vi "arduinoTest.vi"() -> ()   [LabVIEW 2019]
panel:
  out "Timed Out":bool[](array[boolean])
  in  "Commands to Send":T1(array[cluster])=[{"Command"="ST", "Wait For Completion"=TRUE, "Description"="Get status", "Timeout (ms)"=3000.0}, {"Command"="HE", "Wait For Completion"=TRUE, "Description"="Get help", "Timeout (ms)"=3000.0}, {"Command"="CW", "Wait For Completion"=TRUE, "Description"="Get current well", "Timeout (ms)"=3000.0}, {"Command"="FK", "Wait For Completion"=TRUE, "Description"="Bad command to test timeout", "Timeout (ms)"=3000.0}, {"Command"="PSx", "Wait For Completion"=TRUE, "Description"="Get x-axis position", "Timeout (ms)"=3000.0}, {"Command"="PSy", "Wait For Completion"=TRUE, "Description"="get y-axis position", "Timeout (ms)"=3000.0}, {"Command"="TM", "Wait For Completion"=TRUE, "Description"="Test Motor", "Timeout (ms)"=30000.0}, {"Command"="ST", "Wait For Completion"=TRUE, "Description"="Check status", "Timeout (ms)"=3000.0}, {"Command"="FW", "Wait For Completion"=TRUE, "Description"="Gi to first well", "Timeout (ms)"=3000.0}, {"Command"="MO", "Wait For Completion"=TRUE, "Description"="Move to next well", "Timeout (ms)"=3000.0}, {"Command"="ABX1000", "Wait For Completion"=TRUE, "Description"="Absolute move", "Timeout (ms)"=3000.0}, {"Command"="ABY1000", "Wait For Completion"=TRUE, "Description"="Test Motor", "Timeout (ms)"=3000.0}, {"Command"="ABZ1000", "Wait For Completion"=TRUE, "Description"="Test Motor", "Timeout (ms)"=3000.0}, {"Command"="REX1000", "Wait For Completion"=TRUE, "Description"="Test Motor", "Timeout (ms)"=3000.0}, {"Command"="REY1000", "Wait For Completion"=TRUE, "Description"="Test Motor", "Timeout (ms)"=3000.0}, {"Command"="REZ2000", "Wait For Completion"=TRUE, "Description"="Test Motor", "Timeout (ms)"=3000.0}]
  out "Commands Accepted":bool[](array[boolean])
  in  "Wait For Startup (ms)":u32=10000
  out "Recieve Log":string
  out "error out":errorcluster
  in  "Baud Rate":u32=9600
  in  "COM Port":refnum<visa-resource-name>="COM4"
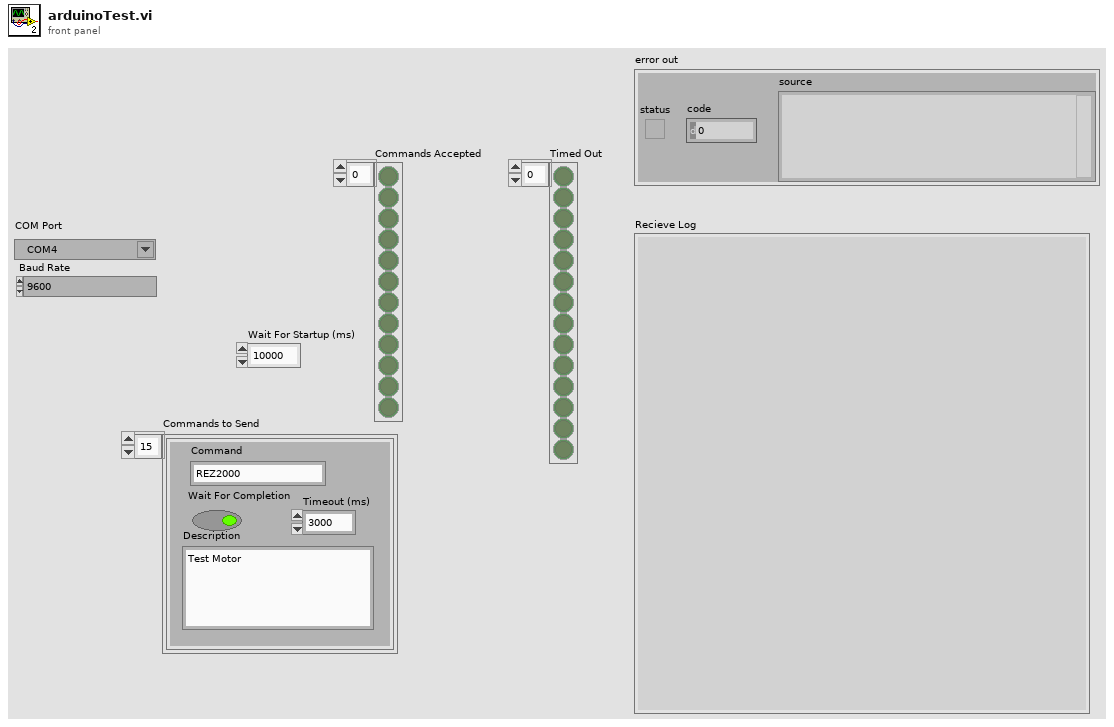
[diagram p1: front panel]
types:
  T1 = cluster{"Command":string, "Wait For Completion":bool, "Description":string, "Timeout (ms)":dbl}[]
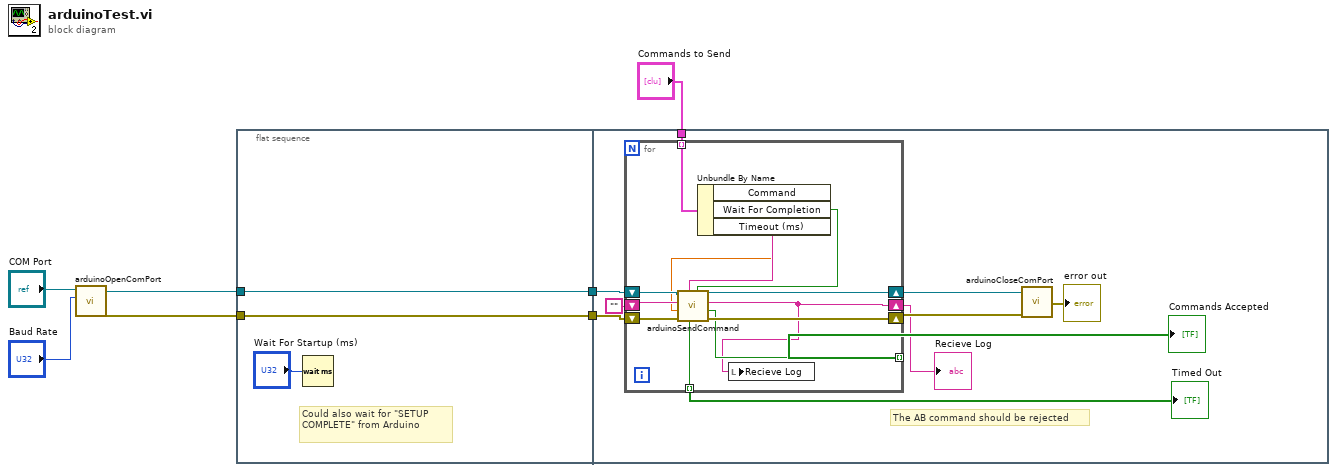
[diagram p0: block diagram]
diagram:
  n1 = call "arduinoOpenComPort.vi"("Baud Rate"="Baud Rate", "COM Port"="COM Port") -> ("error out"=w4:errorcluster, "VISA resource name out"=w5:refnum<visa-resource-name>)  [unwired: 8 in]
  n2 = flat-sequence {
    tunnel: w4 -> [w9]
    tunnel: w5 -> [w10]
    tunnel: [w10] -> w3
    tunnel: [w9] -> w2
    tunnel: w3 -> [w19]
    tunnel: w2 -> [w18]
    tunnel: "Commands to Send" -> [w13]
    frame #0 {
      # "Could also wait for \"SETUP COMPLETE\" from Arduino"
      n3 = Wait (ms)(milliseconds to wait="Wait For Startup (ms)") -> ()  [unwired: 1 out]
    }
    frame #1 {
      # "The AB command should be rejected"
      n4 = for {
        shift-right: [w30] -> w16
        shift-left: w19 -> [w32]
        shift-right: [w29] -> w15
        shift-left: w18 -> [w31]
        shift-right: [w24] -> w12
        shift-left: "" -> [w23]
        tunnel: [w28] -> w14 mode=indexing
        tunnel: w13 -> [w26] mode=indexing
        tunnel: [w22] -> w11 mode=indexing
        n5 = Unbundle By Name(w26) -> ("Command"=w27:string, "Wait For Completion"=w25:bool, "Timeout (ms)"=w21:dbl)
        n6 = call "arduinoSendCommand.vi"("Wait For Completion"=w25, "Input Command"=w27, "error in (no error)"=w31, "Timeout (ms)"=w21, "Input Recieve Log"=w23, "VISA resource name"=w32) -> ("error out"=w29:errorcluster, "Command Accepted"=w28:bool, "Output Recieve Log"=w24:string, "VISA resource name out"=w30:refnum<visa-resource-name>, "Timed Out"=w22:bool)
        n7 = local write "Recieve Log"(w24) -> ()
      }
      "Commands Accepted" <- w14
      "Recieve Log" <- w12
      "Timed Out" <- w11
      n8 = call "arduinoCloseComPort.vi"("Error In"=w15, "VISA resource"=w16) -> ("error out"=→"error out":errorcluster)  [unwired: 9 in]
    }
  }
